vi "Step Script.vi"(6 "Gantry In":refnum<class "Gantry.lvclass">, 7 "Console Log In":refnum<class "Console Log.lvclass">, 8 "error in (no error)":errorcluster, 10 "Pause in":bool, 11 "gScript Interpreter in":refnum<class "gScript Interpreter.lvclass">) -> (0 "error out":errorcluster, 1 "Finished":bool, 2 "Pause out":bool, 3 "gScript Interpreter out":refnum<class "gScript Interpreter.lvclass">, 4 "Gantry Out":refnum<class "Gantry.lvclass">, 5 "Console Log Out":refnum<class "Console Log.lvclass">)   [LabVIEW 2017, in "gScript Interpreter.lvclass"]
uses:
  gScript Interpreter.lvclass
  Application Utilities/Console Log/Console Log.lvclass
  Shared Components/Gantry Class/Gantry.lvclass
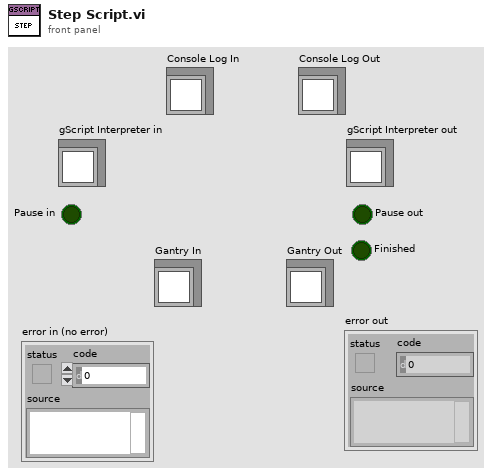
[diagram p1: front panel]
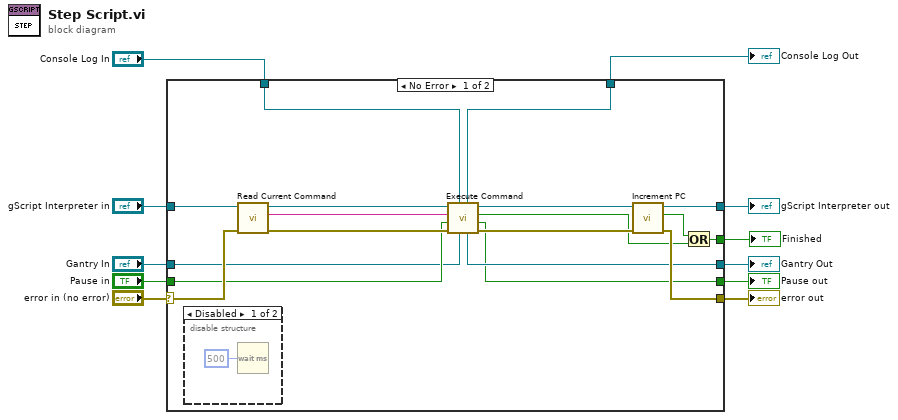
[diagram p0: block diagram]
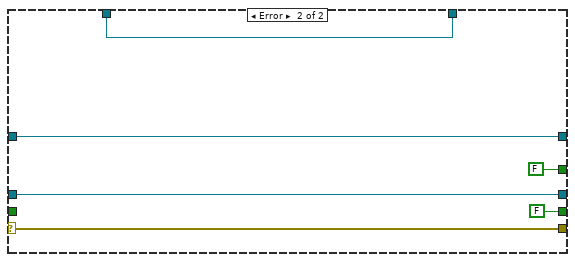
[diagram p3: hidden frame]
diagram:
  n1 = case shown="No Error" "error in (no error)" {
    selector: "error in (no error)" -> [w28 w36]
    tunnel: [w26 w36] -> w10
    tunnel: [w27 w35] -> w8
    tunnel: "gScript Interpreter in" -> [w29 w35]
    tunnel: "Gantry In" -> [w17 w34]
    tunnel: "Console Log In" -> [w25 w33]
    tunnel: [w16 w34] -> w5
    tunnel: [w24 w33] -> w4
    tunnel: [w13 FALSE] -> w3
    tunnel: [w15 FALSE] -> w2
    tunnel: "Pause in" -> [w18 _]
    frame No Error {
      n2 = disable-structure shown="Disabled" {
        frame Disabled {
          n3 = Wait (ms)(milliseconds to wait=u32 500) -> ()  [unwired: 1 out]
        }
        frame Enabled {
        }
      }
      n4 = call-dynamic "Read Current Command.vi"("error in (no error)"=w28, "gScript Interpreter in"=w29) -> ("error out"=w21:errorcluster, "Current Command"=w19:string, "gScript Interpreter out"=w23:refnum<class "gScript Interpreter.lvclass">)  [unwired: 7 in]
      n5 = call-dynamic "Execute Command.vi"("Gantry In"=w17, "Console Log In"=w25, "error in (no error)"=w21, "Pause in"=w18, "Command"=w19, "gScript Interpreter in"=w23) -> ("error out"=w20:errorcluster, "Pause out"=w15:bool, "End out"=w12:bool, "gScript Interpreter out"=w22:refnum<class "gScript Interpreter.lvclass">, "Gantry Out"=w16:refnum<class "Gantry.lvclass">, "Console Log Out"=w24:refnum<class "Console Log.lvclass">)
      n6 = call-dynamic "Increment PC.vi"("error in (no error)"=w20, "gScript Interpreter in"=w22) -> ("error out"=w26:errorcluster, "Finished"=w14:bool, "gScript Interpreter out"=w27:refnum<class "gScript Interpreter.lvclass">)  [unwired: 7 in]
      n7 = Or(x=w14, y=w12) -> (x .or. y?=w13:bool)
    }
    frame Error {
    }
  }
  "error out" <- w10
  "gScript Interpreter out" <- w8
  "Console Log Out" <- w4
  "Gantry Out" <- w5
  "Finished" <- w3
  "Pause out" <- w2
